vi "Disconnect from Slave.vi"(8 "error in":errorcluster, 11 "TCP master in":refnum<class "SMSD.lvclass">) -> (0 "error out":errorcluster, 3 "TCP master out":refnum<class "SMSD.lvclass">)   [LabVIEW 2021, in "SMSD.lvclass"]
doc: "Closes the TCP connection stored in the class."
uses:
  SMSD.lvclass
  SMSD.lvclass/SMSD.ctl
  Master CR.lvclass
  Network Protocol/SMSD Master/SMSD Master.lvclass
  C:/my_projects/projects/Algorithms/Labview/21/Master CR/Master CR.lvclass
  C:/my_projects/projects/Algorithms/Labview/21/Master CR/Devices/SMSD/SMSD.lvclass
  Transmission Data Unit/SMSD/SMSD ADU.lvclass
  C:/my_projects/projects/Algorithms/Labview/21/Modbus_v121c/Network Protocol/Network Protocol.lvclass
  C:/my_projects/projects/Algorithms/Labview/21/Master CR/Network Protocol/SMSD Master/SMSD Master.lvclass
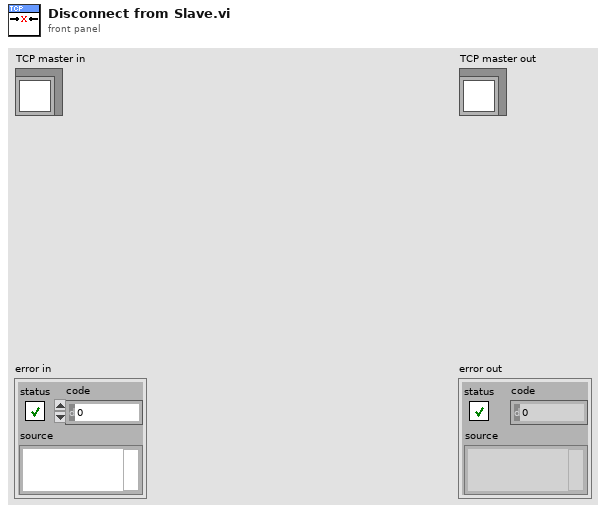
[diagram p1: front panel]
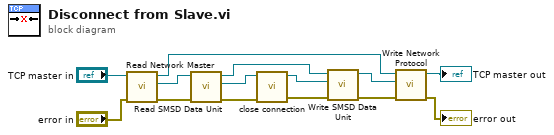
[diagram p0: block diagram]
diagram:
  n1 = call "Read Network Master.vi"("error in (no error)"="error in", "SMSD in"="TCP master in") -> ("error out"=w10:errorcluster, "TCP Master"=w14:refnum<class "SMSD Master.lvclass">, "SMSD out"=w8:refnum<class "SMSD.lvclass">)  [unwired: 7 in]
  n2 = call "Read SMSD Data Unit.vi"("error in (no error)"=w10, "SMSD Master in"=w14) -> ("error out"=w5:errorcluster, "IP Data Unit"=w13:refnum<class "SMSD ADU.lvclass">, "SMSD Master out"=w9:refnum<class "SMSD Master.lvclass">)  [unwired: 7 in]
  n3 = call "close connection.vi"("error in"=w5, "TCP master in"=w13) -> ("error out"=w11:errorcluster, "TCP master out"=w12:refnum<class "SMSD ADU.lvclass">)  [unwired: 8 in]
  n4 = call "Write SMSD Data Unit.vi"("error in (no error)"=w11, "IP Data Unit"=w12, "SMSD Master in"=w9) -> ("error out"=w6:errorcluster, "SMSD Master out"=w7:refnum<class "SMSD Master.lvclass">)  [unwired: 7 in]
  n5 = call "Write Network Protocol.vi"("error in (no error)"=w6, "Network Protocol"=w7, "Master CR in"=w8) -> ("error out"=→"error out":errorcluster, "Master CR out"=→"TCP master out":refnum<class "SMSD.lvclass">)  [unwired: 7 in]
